vi "CDB to JSON Value.vi"(1 "Value":cdb, 2 "Name":string="hello") -> (0 "JSON Value":string)   [LabVIEW 2011, in "LV JSON.lvlib"]
uses:
  LV JSON.lvlib
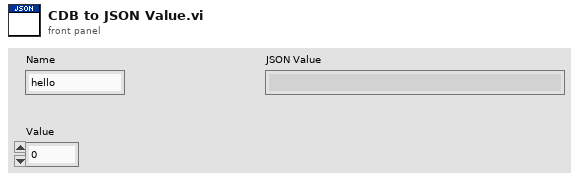
[diagram p1: front panel]
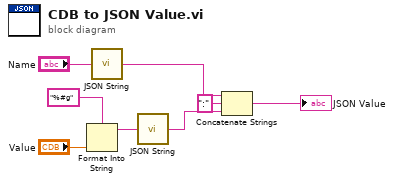
[diagram p0: block diagram]
diagram:
  n1 = Format Into String(format string="%#g", "Value") -> (resulting string=w2:string)  [unwired: 2 in, 1 out]
  n2 = call "JSON String.vi"("in"="Name") -> ("out"=w7:string)
  n3 = call "JSON String.vi"("in"=w2) -> ("out"=w1:string)
  n4 = Concatenate Strings(w7, ":" ("string"), w1) -> (→"JSON Value":string)
